vi "Add to Map.vi"(6 "Parent (None)":string[](array[string]), 7 "Name Prefix (None)":string, 9 "Channel (Not Channel)":T1, 10 "Name":string, 11 "Map in":map{string[], T2}(c390)) -> (3 "Map":map{string[], T2}(c390), 4 "Hierarchy":string[](array[string]))   [LabVIEW 2020, in "VolatusDAQGenericGUI.lvlib"]
uses:
  VolatusDAQGenericGUI.lvlib
  AI Tree Entry.ctl
  Channel Entry.ctl
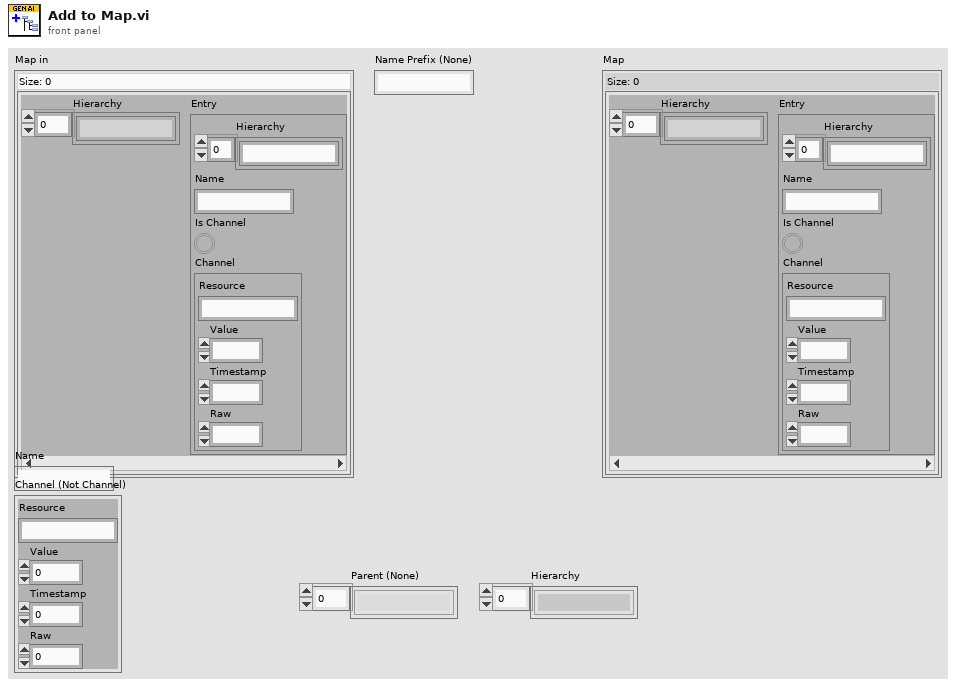
[diagram p1: front panel]
types:
  T1 = typedef "VolatusDAQGenericGUI.lvlib/Channel Entry.ctl" = cluster{"Resource":string, "Value":dbl, "Timestamp":dbl, "Raw":dbl}
  T2 = typedef "VolatusDAQGenericGUI.lvlib/AI Tree Entry.ctl" = cluster{"Hierarchy":string[], "Name":string, "Is Channel":bool, "Channel":T1}
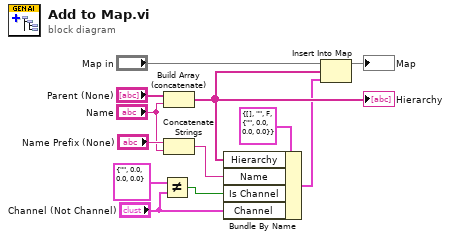
[diagram p0: block diagram]
diagram:
  n1 = Not Equal?(x=T1 {"Resource"="", "Value"=0.0, "Timestamp"=0.0, "Raw"=0.0}, y="Channel (Not Channel)") -> (x != y?=w6:bool)
  n2 = Build Array (concatenate)("Parent (None)", "Name") -> (w2:string[])
  "Hierarchy" <- w2
  n3 = Concatenate Strings("Name Prefix (None)", "Name") -> (w5:string)
  n4 = Bundle By Name(cluster=T2 {"Hierarchy"=[], "Name"="", "Is Channel"=FALSE, "Channel"={"Resource"="", "Value"=0.0, "Timestamp"=0.0, "Raw"=0.0}} ("AI Tree Entry"), "Hierarchy"=w2, "Name"=w5, "Is Channel"=w6, "Channel"="Channel (Not Channel)") -> (w1:T2)
  n5 = Insert Into Map(map in="Map in", key=w2, value=w1) -> (map out=→"Map":map{string[], T2})  [unwired: 2 out]
